vi "Compute IRF(X)PSED Fitted Plot.vi"(8 "error in (no error)":errorcluster, 9 "IRF*PSED Fit Parameters":T1, 10 "Original Plot":cluster{"X Array":dbl[], "Y Array":dbl[]}, 11 "Ramp Pattern":dbl[](array[numeric])) -> (0 "error out":errorcluster, 2 "Fitted Plot":cluster{"X Array":dbl[], "Y Array":dbl[]})   [LabVIEW 2019]
uses:
  IRF(X)PSED Fit Parameters.ctl
  IRF(X)PSED Fixed Parameters v3.ctl
  IRF(X)PSED Extraction Options.ctl
  Fourier Series Smoothing Option.ctl
  Fourier Series Truncation.ctl
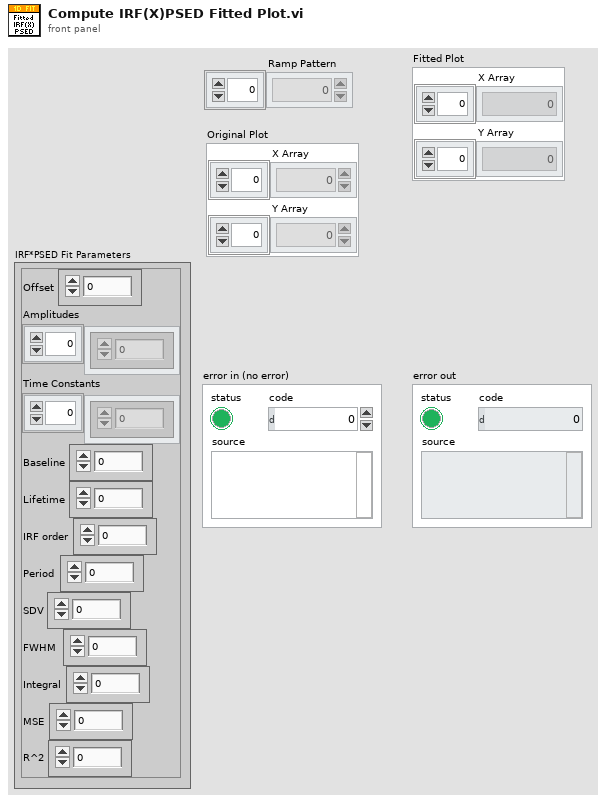
[diagram p1: front panel]
types:
  T1 = typedef "IRF(X)PSED Fit Parameters.ctl" = cluster{"Offset":dbl, "Amplitudes":dbl[], "Time Constants":dbl[], "Baseline":dbl, "Lifetime":dbl, "IRF order":dbl, "Period":dbl, "SDV":dbl, "FWHM":dbl, "Integral":dbl, "MSE":dbl, "R^2":dbl}
  T2 = typedef "IRF(X)PSED Fixed Parameters v3.ctl" = cluster{"order":i32, "T":dbl, "Time Constant Array":dbl[], "{S_k, C_k, phi_k, e_k} arrays":cluster{"S_k Array":dbl[], "C_k Array":dbl[], "phi_k Array":dbl[], "e_k Array":dbl[]}, "IRF Extraction Options":T3}
  T3 = typedef "IRF(X)PSED Extraction Options.ctl" = cluster{"Time Constant for IRF Extraction":dbl[unit], "IRF Order":i32, "Fourier Series Smoothing":T4, "Noise Threshold":dbl, "Smoothing Width":dbl, "Fourier Series Truncation":T5, "Truncation Order":i32, "Save Power Spectrum":bool}
  T4 = typedef "Fourier Series Smoothing Option.ctl" = enum16{"None", "Lanczos Factors", "Fejer Summation"}
  T5 = typedef "Fourier Series Truncation.ctl" = enum16{"Automatic", "Fixed"}
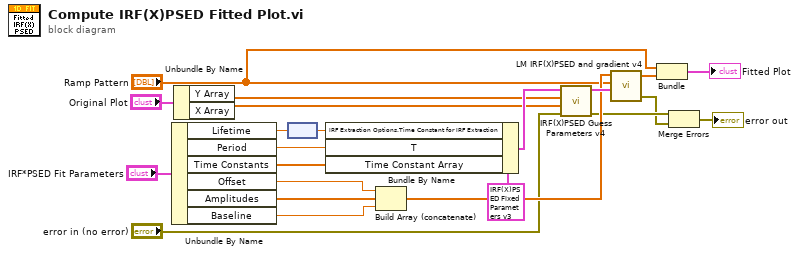
[diagram p0: block diagram]
diagram:
  n1 = Unbundle By Name("IRF*PSED Fit Parameters") -> ("Lifetime"=w16:dbl, "Period"=w17:dbl, "Time Constants"=w19:dbl[], "Offset"=w12:dbl, "Amplitudes"=w20:dbl[], "Baseline"=w13:dbl)
  n2 = Unbundle By Name("Original Plot") -> ("Y Array"=w6:dbl[], "X Array"=w7:dbl[])
  n3 = node(w16) -> (w21:dbl[unit])
  n4 = Bundle By Name(cluster=T2 {"order"=0, "T"=0.0, "Time Constant Array"=[], "{S_k, C_k, phi_k, e_k} arrays"={"S_k Array"=[], "C_k Array"=[], "phi_k Array"=[], "e_k Array"=[]}, "IRF Extraction Options"={"Time Constant for IRF Extraction"=1e-18, "IRF Order"=0, "Fourier Series Smoothing"=enum."None", "Noise Threshold"=0.0, "Smoothing Width"=0.0, "Fourier Series Truncation"=enum."Automatic", "Truncation Order"=0, "Save Power Spectrum"=FALSE}} ("IRF*PSED fixed Parameters"), "IRF Extraction Options.Time Constant for IRF Extraction"=w21, "T"=w17, "Time Constant Array"=w19) -> (w18:T2)
  n5 = Build Array (concatenate)(w12, w20, w13) -> (w14:dbl[])
  n6 = call "IRF(X)PSED Guess Parameters v4.vi"("Error In"="error in (no error)", "X Array"=w7, "Y Array"=w6, "IRF*PSED fixed Parameters (in)"=w18) -> ("Error Out"=w3:errorcluster, "IRF*PSED fixed Parameters (out)"=w22:T2)  [unwired: 3 in, 3 out]
  n7 = call "LM IRF(X)PSED and gradient v4.vi"("data"=w22, "X"="Ramp Pattern", "a"=w14) -> ("error out"=w2:errorcluster, "f(X,a)"=w11:dbl[])  [unwired: 1 in, 1 out]
  n8 = Bundle("Ramp Pattern"="Ramp Pattern", "f(X,a)"=w11) -> (→"Fitted Plot":cluster{"Ramp Pattern":dbl[], "f(X,a)":dbl[]})  [unwired: 1 in]
  n9 = Merge Errors(w3, w2) -> (→"error out":errorcluster)
